vi "Split Operator & Operand.vi"(3 "Operation":string) -> (0 "Operand":string, 1 "Operator":string)   [LabVIEW 2020, in "AoC 2022.lvlib"]
uses:
  AoC 2022.lvlib
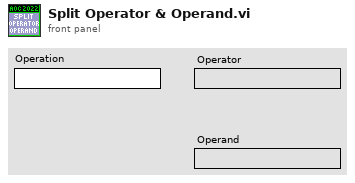
[diagram p1: front panel]
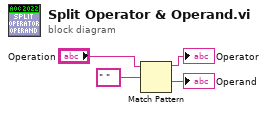
[diagram p0: block diagram]
diagram:
  n1 = Match Pattern(string="Operation", regular expression=" ") -> (before substring=→"Operator":string, after substring=→"Operand":string)  [unwired: 1 in, 2 out]
